vi "accumulator tests.vi"() -> ()   [LabVIEW 2014]
uses:
  <vilib>/Rock Robotics/WPI/Gyro/WPI_GyroDevRef.ctl
  <vilib>/Rock Robotics/SystemInterfaces/Typedef/FPGA_TypedefAnalogModule.ctl
  <vilib>/Rock Robotics/SystemInterfaces/AI/FPGA_AIChannel.ctl
  <vilib>/Rock Robotics/SystemInterfaces/Typedef/FPGA_TypedefAnalogModuleForGyro.ctl
  <vilib>/Rock Robotics/SystemInterfaces/AI/FPGA_AIGyroChannel.ctl
  <vilib>/Rock Robotics/WPI/AnalogChannel/WPI_AnalogChannelDevRef.ctl
  <vilib>/Rock Robotics/SystemInterfaces/AI/FPGA_AIDevRef.ctl
  <vilib>/Rock Robotics/SystemInterfaces/System/FPGA_SystemGet.vi
  <vilib>/Rock Robotics/SystemInterfaces/AI/FPGA_ReadAI.vi
panel:
  in  "Reset":bool
  out "Angular Rate Max":dbl
  out "Calibrate Loop":bool
  out "Angle 2":dbl(knob) scale=0.0..360.0
  in  "Disabled":bool
  out "Angular Rate":dbl
  out "error out":errorcluster
  out "Angle":dbl
  out "GyroDevRef":T1={"DevStatus"={"status"=FALSE, "code"=0, "source"=""}, "Analog Module"=enum."Controller 1", "Analog Channel"=enum."AI 1", "Offset"=0.0, "Gain (VoltsPerDegree/Second)"=0.0}
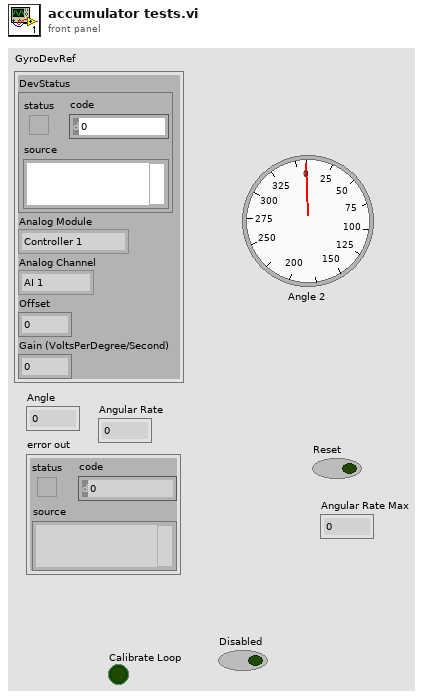
[diagram p1: front panel]
types:
  T1 = typedef "WPI_GyroDevRef.ctl" = cluster{"DevStatus":errorcluster, "Analog Module":T2, "Analog Channel":T3, "Offset":dbl, "Gain (VoltsPerDegree/Second)":dbl}
  T2 = typedef "FPGA_TypedefAnalogModule.ctl" = enum16{"Controller 1"}
  T3 = typedef "FPGA_AIChannel.ctl" = enum8{"AI 0", "AI 1", "AI 2", "AI 3", "AI MXP 0", "AI MXP 1", "AI MXP 2", "AI MXP 3", "Invalid"}
  T4 = typedef "WPI_AnalogChannelDevRef.ctl" = cluster{"DevStatus":errorcluster, "Controller":T2, "Analog Channel":T3}
  T5 = typedef "FPGA_AIGyroChannel.ctl" = enum8{"AI 0", "AI 1", "Invalid"}
  T6 = typedef "FPGA_TypedefAnalogModuleForGyro.ctl" = enum16{"Controller 1"}
  T7 = typedef "FPGA_AIDevRef.ctl" = cluster{"DevStatus":errorcluster, "Controller":T2}
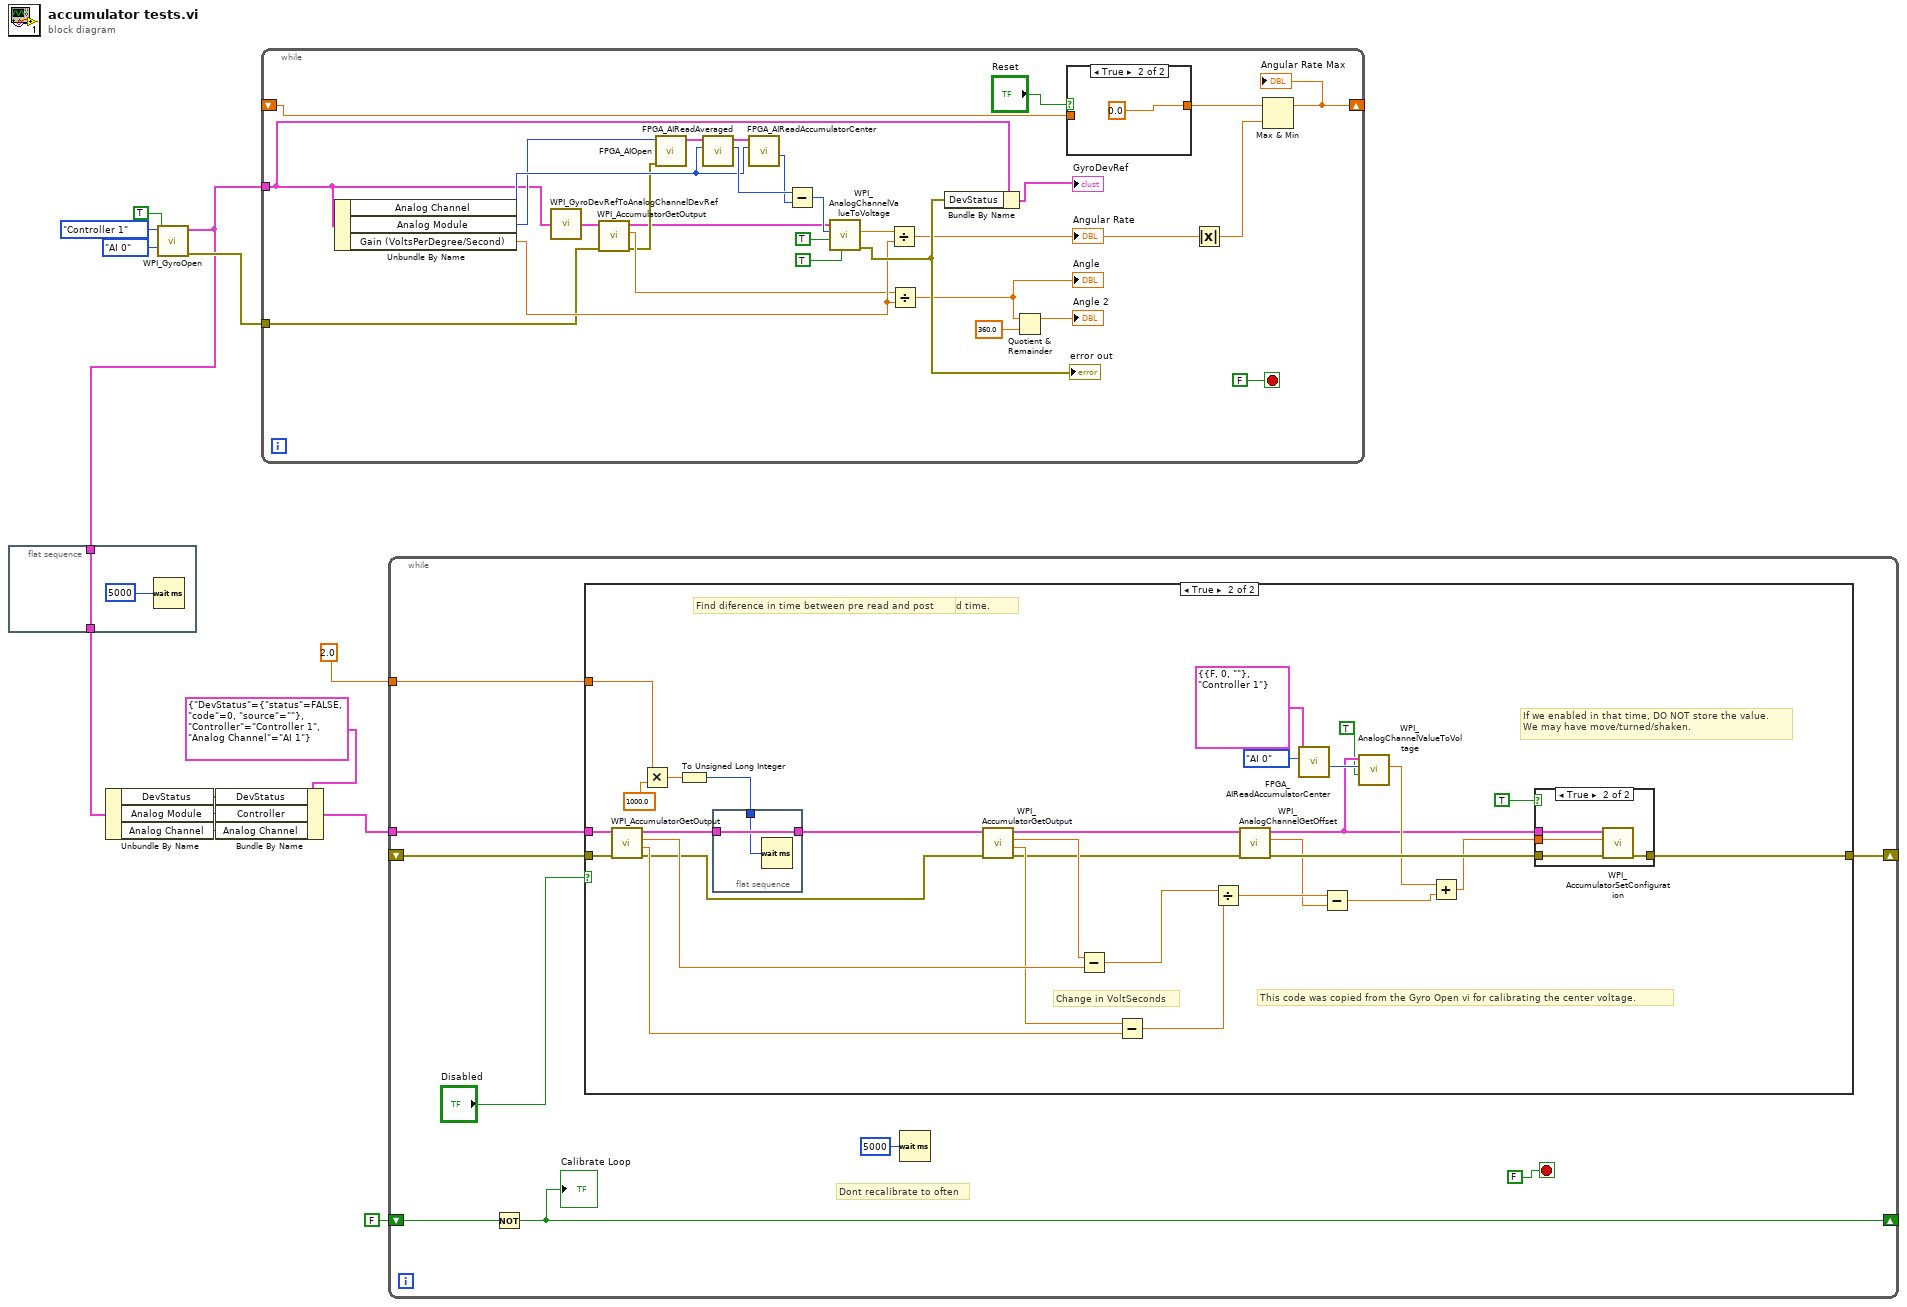
[diagram p0: block diagram]
diagram:
  n1 = flat-sequence {
    tunnel: w2 -> [w15]
    tunnel: [w15] -> w1
    frame #0 {
      n2 = Wait (ms)(milliseconds to wait=u32 5000) -> ()  [unwired: 1 out]
    }
  }
  n3 = Unbundle By Name(w1) -> ("DevStatus"=w5:errorcluster, "Analog Module"=w4:T2, "Analog Channel"=w3:T3)
  n4 = call <vilib>:"WPI_GyroOpen.vi"("Calibrate On Open"=TRUE, "Analog Channel"=FPGA_AIGyroChannel."AI 0", "Controller"=FPGA_TypedefAnalogModuleForGyro."Controller 1") -> ("error out"=w13:errorcluster, "GyroDevRef"=w2:T1)  [unwired: 6 in, 1 out]
  n5 = Bundle By Name(cluster=T4 {"DevStatus"={"status"=FALSE, "code"=0, "source"=""}, "Controller"=enum."Controller 1", "Analog Channel"=enum."AI 1"} ("AIDeviceRef"), "DevStatus"=w5, "Controller"=w4, "Analog Channel"=w3) -> (w8:T4)
  n6 = while {
    tunnel: w2 -> [w27]
    tunnel: w13 -> [w26]
    shift-right: [w19] -> _
    shift-left: _ -> [w18]
    stop <- FALSE stop-if-true
    n7 = Unbundle By Name(w27) -> ("Analog Channel"=w38:T3, "Analog Module"=w28:T2, "Gain (VoltsPerDegree/Second)"=w37:dbl)
    n8 = call <vilib>:"WPI_GyroDevRefToAnalogChannelDevRef.vi"("GyroDeviceRef"=w27) -> ("AIDeviceRef"=w42:T4)  [unwired: 4 out]
    n9 = call <vilib>:"WPI_AccumulatorGetOutput.vi"("error in (no error)"=w26, "AIDeviceRef"=w42) -> ("error out"=w34:errorcluster, "Value (Volt Seconds)"=w36:dbl, "AIDeviceRef"=w29:T4)  [unwired: 7 out]
    n10 = call <vilib>:"FPGA_AIOpen.vi"("error in (no error)"=w34, "Controller"=w28) -> ("AI Reference out"=w35:T7)  [unwired: 1 in, 8 out]
    n11 = call <vilib>:"FPGA_AIReadAveraged.vi"("Channel"=w38, "AI Reference in"=w35) -> ("Averaged"=w41:i32, "AI Reference out"=w40:T7)  [unwired: 1 in, 7 out]
    n12 = call <vilib>:"FPGA_AIReadAccumulatorCenter.vi"("Channel"=w38, "AI Reference in"=w40) -> ("Center"=w39:i32)  [unwired: 1 in, 8 out]
    n13 = Subtract(x=w41, y=w39) -> (x-y=w33:i32)
    n14 = call <vilib>:"WPI_AnalogChannelValueToVoltage.vi"("Relative"=TRUE, "Averaged"=TRUE, "Value"=w33, "AIDeviceRef"=w29) -> ("error out"=w43:errorcluster, "Voltage"=w31:dbl)  [unwired: 1 in, 5 out]
    "error out" <- w43
    n15 = Divide(x=w31, y=w37) -> (x/y=w21:dbl)
    "Angular Rate" <- w21
    n16 = Divide(x=w36, y=w37) -> (x/y=w24:dbl)
    "Angle" <- w24
    n17 = Bundle By Name(cluster=w27, "DevStatus"=w43) -> (→"GyroDevRef":T1)
    n18 = Quotient & Remainder(x=w24, y=360.0) -> (x-y*floor(x/y)=→"Angle 2":dbl)  [unwired: 1 out]
    n19 = case shown="True" "Reset" {
      tunnel: w18 -> [w45 _]
      tunnel: [w45 0.0] -> w17
      frame False {
      }
      frame True {
      }
    }
    n20 = Absolute Value(x=w21) -> (abs(x)=w20:dbl)
    n21 = Max & Min(x=w17, y=w20) -> (max(x,y)=w19:dbl)  [unwired: 1 out]
    "Angular Rate Max" <- w19
  }
  n22 = while {
    tunnel: 2.0 ("Calibration Time (s)") -> [w54]
    tunnel: w8 -> [w55]
    shift-right: [w53] -> _
    shift-left: _ -> [w52]
    shift-right: [w47] -> _
    shift-left: FALSE -> [w48]
    stop <- FALSE stop-if-true
    # "Dont recalibrate to often"
    n23 = Not(x=w48) -> (.not. x?=w47:bool)
    "Calibrate Loop" <- w47
    n24 = case shown="True" "Disabled" {
      tunnel: w54 -> [_ w86]
      tunnel: w55 -> [_ w79]
      tunnel: [w56 w66] -> w53
      tunnel: w52 -> [w56 w80]
      frame False {
      }
      frame True {
        # "Change in VoltSeconds"
        # "Find diference in time between pre read and post"
        # "Make sure to get robot mode after waiting for specified time."
        # "This code was copied from the Gyro Open vi for calibrating the center voltage."
        # "If we enabled in that time, DO NOT store the value.\nWe may have move/turned/shaken."
        n25 = call <vilib>:"WPI_AccumulatorGetOutput.vi"("error in (no error)"=w80, "AIDeviceRef"=w79) -> ("error out"=w68:errorcluster, "Duration (Seconds)"=w78:dbl, "Value (Volt Seconds)"=w77:dbl, "AIDeviceRef"=w81:T4)  [unwired: 6 out]
        n26 = Multiply(x=w86, y=1000.0) -> (x*y=w83:dbl)
        n27 = To Unsigned Long Integer(number=w83) -> (unsigned 32bit integer=w82:u32)
        n28 = flat-sequence {
          tunnel: w81 -> [w93]
          tunnel: w82 -> [w92]
          tunnel: [w93] -> w67
          frame #0 {
            n29 = Wait (ms)(milliseconds to wait=w92) -> ()  [unwired: 1 out]
          }
        }
        n30 = call <vilib>:"WPI_AccumulatorGetOutput.vi"("error in (no error)"=w68, "AIDeviceRef"=w67) -> ("error out"=w69:errorcluster, "Duration (Seconds)"=w74:dbl, "Value (Volt Seconds)"=w76:dbl, "AIDeviceRef"=w72:T4)  [unwired: 6 out]
        n31 = Subtract(x=w76, y=w77) -> (x-y=w75:dbl)
        n32 = Subtract(x=w74, y=w78) -> (x-y=w73:dbl)
        n33 = Divide(x=w75, y=w73) -> (x/y=w85:dbl)
        n34 = call <vilib>:"WPI_AnalogChannelGetOffset.vi"("error in (no error)"=w69, "AIDeviceRef"=w72) -> ("error out"=w71:errorcluster, "Offset"=w70:dbl, "AIDeviceRef"=w58:T4)  [unwired: 7 out]
        n35 = call <vilib>:"FPGA_AIReadAccumulatorCenter.vi"("Channel"=FPGA_AIChannel."AI 0", "AI Reference in"=T7 {"DevStatus"={"status"=FALSE, "code"=0, "source"=""}, "Controller"=enum."Controller 1"}) -> ("Center"=w60:i32)  [unwired: 7 in, 2 out]
        n36 = Subtract(x=w85, y=w70) -> (x-y=w62:dbl)
        n37 = call <vilib>:"WPI_AnalogChannelValueToVoltage.vi"("Averaged"=TRUE, "Value"=w60, "AIDeviceRef"=w58) -> ("Voltage"=w59:dbl)  [unwired: 6 in, 2 out]
        n38 = Add(x=w59, y=w62) -> (x+y=w61:dbl)
        n39 = case shown="True" TRUE {
          tunnel: [w87 w91] -> w66
          tunnel: w71 -> [w87 w90]
          tunnel: w61 -> [_ w88]
          tunnel: w58 -> [_ w89]
          frame False {
          }
          frame True {
            n40 = call <vilib>:"WPI_AccumulatorSetConfiguration.vi"("error in (no error)"=w90, "Center"=w88, "AIDeviceRef"=w89) -> ("error out"=w91:errorcluster)  [unwired: 2 in, 6 out]
          }
        }
      }
    }
    n41 = Wait (ms)(milliseconds to wait=u32 5000) -> ()  [unwired: 1 out]
  }
